vi "Get HOST Serial Port Parameters.vi"(0 "VISA resource name":refnum<visa-resource-name>, 11 "error in (no error)":errorcluster) -> (2 "Baud Rate":i32, 3 "Interface":i32, 4 "VISA resource name out":refnum<visa-resource-name>, 6 "Flow Control":i32, 8 "Number Data Bits":i32, 10 "Number Stop Bits":i32, 13 "End of Line Char":i32, 14 "Parity":i32, 15 "error out":errorcluster)   [LabVIEW 2011, in "Fluke 5XXX Series Multicalibrators.lvlib"]
doc: "This VI returns the RS-232-C settings for the Calibrator rear panel SERIAL 1 FROM HOST serial port."
uses:
  Fluke 5XXX Series Multicalibrators.lvlib
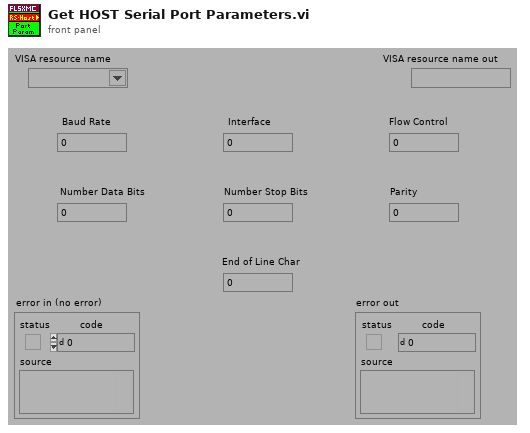
[diagram p1: front panel]
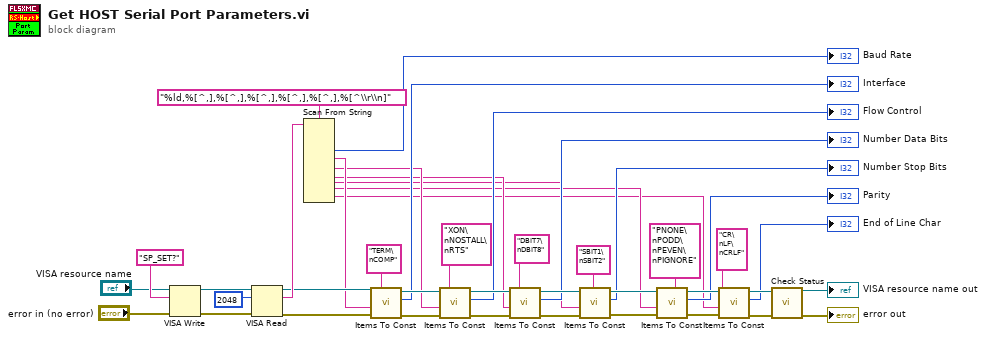
[diagram p0: block diagram]
diagram:
  n1 = VISA Write(VISA resource name="VISA resource name", write buffer="SP_SET?", error in (no error)="error in (no error)") -> (VISA resource name out=w42:refnum<visa-resource-name>, error out=w41:errorcluster)  [unwired: 1 out]
  n2 = VISA Read(VISA resource name=w42, byte count=u32 2048 ("byte count (0)"), error in (no error)=w41) -> (VISA resource name out=w28:refnum<visa-resource-name>, read buffer=w38:string, error out=w35:errorcluster)  [unwired: 1 out]
  n3 = Scan From String(format string="%ld,%[^,],%[^,],%[^,],%[^,],%[^,],%[^\\r\\n]", input string=w38) -> (output 1=→"Baud Rate":i32, output 2=w19:string, output 3=w16:string, output 4=w13:string, output 5=w10:string, output 6=w7:string, output 7=w2:string)  [unwired: 9 in, 3 out]
  n4 = call "Items To Const.vi"("error in (no error)"=w35, "String Item"=w19, "Multi-Line String"="TERM\nCOMP" ("Reset Command"), "VISA resource name"=w28) -> ("error out"=w34:errorcluster, "Index"=→"Interface":i32, "VISA resource name out"=w27:refnum<visa-resource-name>)  [unwired: 5 in]
  n5 = call "Items To Const.vi"("error in (no error)"=w34, "String Item"=w16, "Multi-Line String"="XON\nNOSTALL\nRTS" ("Reset Command"), "VISA resource name"=w27) -> ("error out"=w33:errorcluster, "Index"=→"Flow Control":i32, "VISA resource name out"=w26:refnum<visa-resource-name>)  [unwired: 5 in]
  n6 = call "Items To Const.vi"("error in (no error)"=w33, "String Item"=w13, "Multi-Line String"="DBIT7\nDBIT8" ("Reset Command"), "VISA resource name"=w26) -> ("error out"=w32:errorcluster, "Index"=→"Number Data Bits":i32, "VISA resource name out"=w25:refnum<visa-resource-name>)  [unwired: 5 in]
  n7 = call "Items To Const.vi"("error in (no error)"=w32, "String Item"=w10, "Multi-Line String"="SBIT1\nSBIT2" ("Reset Command"), "VISA resource name"=w25) -> ("error out"=w31:errorcluster, "Index"=→"Number Stop Bits":i32, "VISA resource name out"=w24:refnum<visa-resource-name>)  [unwired: 5 in]
  n8 = call "Items To Const.vi"("error in (no error)"=w31, "String Item"=w7, "Multi-Line String"="PNONE\nPODD\nPEVEN\nPIGNORE" ("Reset Command"), "VISA resource name"=w24) -> ("error out"=w30:errorcluster, "Index"=→"Parity":i32, "VISA resource name out"=w23:refnum<visa-resource-name>)  [unwired: 5 in]
  n9 = call "Items To Const.vi"("error in (no error)"=w30, "String Item"=w2, "Multi-Line String"="CR\nLF\nCRLF" ("Reset Command"), "VISA resource name"=w23) -> ("error out"=w5:errorcluster, "Index"=→"End of Line Char":i32, "VISA resource name out"=w4:refnum<visa-resource-name>)  [unwired: 5 in]
  n10 = call "Check Status.vi"("VISA resource name"=w4, "error in (no error)"=w5) -> ("VISA resource name out"=→"VISA resource name out":refnum<visa-resource-name>, "error out"=→"error out":errorcluster)  [unwired: 12 in]
